vi "CSTK_BuildApplication_Manager_getSetting.vi"(8 "Error in":errorcluster caption="错误输入") -> (0 "Error out":errorcluster caption="错误输出", 2 "BuildApplication Selector":T1={"Package as a ZIP file?"=TRUE, "Rename EXE File Name?"=FALSE}, 3 "Setting path":path)   [LabVIEW 2015, in "CSTK_BuildApplication_Manager.lvlib"]
uses:
  CSTK_BuildApplication_Manager.lvlib
  CSTK_BuildApplication_Manager_selector.ctl
  <vilib>/addons/_JKI.lib/Serialization/JSON/JKI JSON Serialization.lvlib
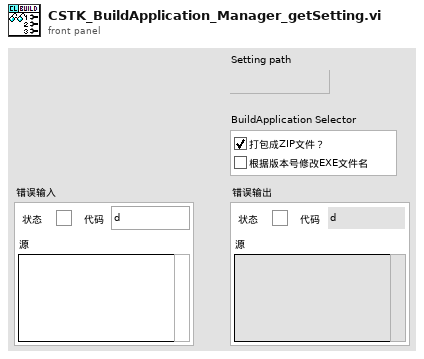
[diagram p1: front panel]
types:
  T1 = typedef "CSTK_BuildApplication_Manager.lvlib/CSTK_BuildApplication_Manager_selector.ctl" = cluster{"Package as a ZIP file?":bool, "Rename EXE File Name?":bool}
  T2 = enum16{"open", "replace", "create", "open or create", "replace or create", "replace or create with confirmation"}
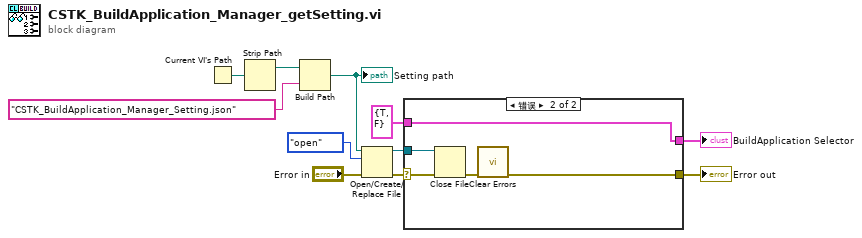
[diagram p0: block diagram]
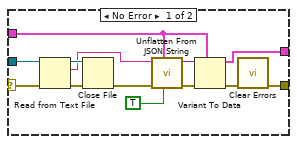
[diagram p2: hidden frame]
diagram:
  n1 = Current VI's Path() -> (path=w11:path)
  n2 = Strip Path(path=w11) -> (stripped path=w10:path)  [unwired: 1 out]
  n3 = Build Path(base path=w10, name or relative path="CSTK_BuildApplication_Manager_Setting.json" ("名称或相对路径")) -> (appended path=w1:path)
  "Setting path" <- w1
  n4 = Open/Create/Replace File(file path (use dialog)=w1, error in="Error in", operation (0:open)=T2."open" ("操作(0:open)")) -> (refnum out=w5:refnum<file>, error out=w6:errorcluster)  [unwired: 3 in, 1 out]
  n5 = case shown="错误" w6 {
    selector: w6 -> [w23 w26]
    tunnel: w5 -> [w24 w27]
    tunnel: [w12 w28] -> w4
    tunnel: [w15 w29] -> w3
    tunnel: T1 {"Package as a ZIP file?"=TRUE, "Rename EXE File Name?"=FALSE} ("BuildApplication Selector") -> [w14 w29]
    frame No Error {
      n6 = Read from Text File(file (use dialog)=w24, error in=w23) -> (refnum out=w22:refnum<file>, text=w20:string, error out=w21:errorcluster)  [unwired: 2 in, 1 out]
      n7 = Close File(refnum=w22, error in=w21) -> (error out=w19:errorcluster)  [unwired: 1 out]
      n8 = call <vilib>:"Unflatten From JSON String.vi"("Nulls as Defaults (F)"=TRUE, "Type and Defaults"=w14, "error in (no error)"=w19, "JSON String"=w20) -> ("error out"=w17:errorcluster, "Variant"=w16:variant)  [unwired: 6 in]
      n9 = Variant To Data(error in=w17, type=w14, Variant=w16) -> (data=w15:T1, error out=w13:errorcluster)
      n10 = call <vilib>:"Clear Errors.vi"("error in (no error)"=w13) -> ("error out"=w12:errorcluster)  [unwired: 5 in, 1 out]
    }
    frame Error {
      n11 = Close File(refnum=w27, error in=w26) -> (error out=w25:errorcluster)  [unwired: 1 out]
      n12 = call <vilib>:"Clear Errors.vi"("error in (no error)"=w25) -> ("error out"=w28:errorcluster)  [unwired: 5 in, 1 out]
    }
  }
  "Error out" <- w4
  "BuildApplication Selector" <- w3
